vi "Read IFD Entry.vi"(3 "Litt/BigEnd":bool, 4 "Directory Offset in":i32, 5 "Image Data in":u8[](array[numeric])) -> (0 "Cluster":T1, 1 "Next Directory Offset Out\n(IN + 12)":i32, 2 "Image Data Out":u8[](array[numeric]))   [LabVIEW 2015, in "Tiff reader.lvlib"]
doc: "Reads the next tag entry in the Image File Directory in a tiff file byte stream, returning the tag, its format and location in the byte stream."
uses:
  Tiff reader.lvlib
  IFD Entry.ctl
  FieldTypes.ctl
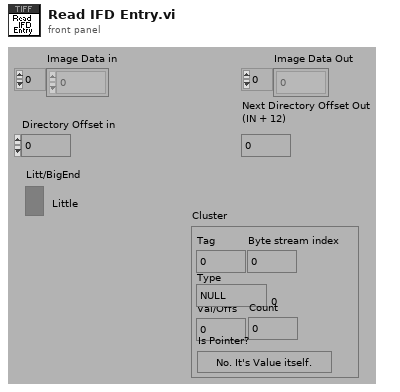
[diagram p1: front panel]
types:
  T1 = typedef "Tiff reader.lvlib/IFD Entry.ctl" = cluster{"Tag":u16, "Type":T2, "Count":u32, "Val/Offs":u32, "Is Pointer?":bool, "Byte stream index":i32}
  T2 = typedef "Tiff reader.lvlib/FieldTypes.ctl" = enum16{"NULL", "U8", "ASCII7", "U16", "U32", "RATIONAL", "SByte(I8)", "Undef(8Bit)", "I16", "I32", "SRat(4B:4B)", "SGL(4Byte)", "DBL(8Byte)"}
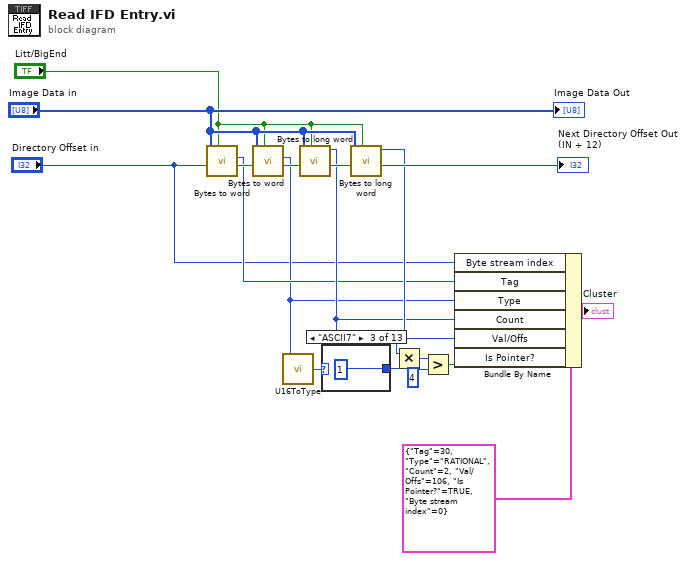
[diagram p0: block diagram]
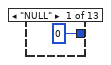
[diagram p2: hidden frame]
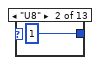
[diagram p3: hidden frame]
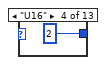
[diagram p4: hidden frame]
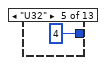
[diagram p5: hidden frame]
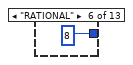
[diagram p6: hidden frame]
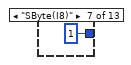
[diagram p7: hidden frame]
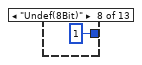
[diagram p8: hidden frame]
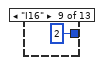
[diagram p9: hidden frame]
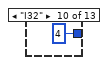
[diagram p10: hidden frame]
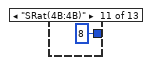
[diagram p11: hidden frame]
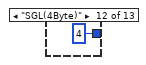
[diagram p12: hidden frame]
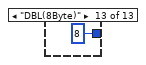
[diagram p13: hidden frame]
diagram:
  n1 = call "Bytes to word.vi"("Litt/BigEnd"="Litt/BigEnd", "Index"="Directory Offset in", "Image Data in"="Image Data in") -> ("Index+2"=w16:i32, "Word"=w4:u16)  [unwired: 1 in, 4 out]
  n2 = call "Bytes to word.vi"("Litt/BigEnd"="Litt/BigEnd", "Index"=w16, "Image Data in"="Image Data in") -> ("Index+2"=w15:i32, "Word"=w3:u16)  [unwired: 1 in, 4 out]
  n3 = call "U16ToType.vi"("U16 In"=w3) -> ("Type out"=w11:T2)  [unwired: 4 out]
  n4 = call "Bytes to long word.vi"("Litt/BigEnd"="Litt/BigEnd", "Index"=w15, "Image Data in"="Image Data in") -> ("Index+4"=w14:i32, "U32"=w9:u32)  [unwired: 5 out]
  n5 = case shown="\"ASCII7\"" w11 {
    tunnel: [i64 0 i64 1 i64 1 i64 2 i64 4 i64 8 i64 1 i64 1 i64 2 i64 4 i64 8 i64 4 i64 8] -> w10
    frame "NULL" {
    }
    frame "U8" {
    }
    frame "ASCII7" {
    }
    frame "U16" {
    }
    frame "U32" {
    }
    frame "RATIONAL" {
    }
    frame "SByte(I8)" {
    }
    frame "Undef(8Bit)" {
    }
    frame "I16" {
    }
    frame "I32" {
    }
    frame "SRat(4B:4B)" {
    }
    frame "SGL(4Byte)" {
    }
    frame "DBL(8Byte)" {
    }
  }
  n6 = call "Bytes to long word.vi"("Litt/BigEnd"="Litt/BigEnd", "Index"=w14, "Image Data in"="Image Data in") -> ("Index+4"=→"Next Directory Offset Out\n(IN + 12)":i32, "U32"=w12:u32)  [unwired: 5 out]
  n7 = Multiply(x=w9, y=w10) -> (x*y=w8:i64)
  n8 = Greater?(x=w8, y=i64 4) -> (0:w6:bool)
  n9 = Bundle By Name(cluster=T1 {"Tag"=30, "Type"=enum."RATIONAL", "Count"=2, "Val/Offs"=106, "Is Pointer?"=TRUE, "Byte stream index"=0} ("Cluster"), "Byte stream index"="Directory Offset in", "Tag"=w4, "Type"=w3, "Count"=w9, "Val/Offs"=w12, "Is Pointer?"=w6) -> (→"Cluster":T1)
  "Image Data Out" <- "Image Data in"
